vi "Configure Output.vi"(6 "Output Type  (0: Sweeping)":i32(ring) items=["Sweeping", "Measuring", "Main Trigger", "Gate Trigger", "Gate", "Odd/Even Trace Point", "Off"], 8 "error in (no error)":errorcluster, 9 "Trigger Polarity  (0: Positive)":i32(ring) items=["Positive", "Negative"], 10 "Trigger Out  (0: Trigger1)":i32(ring) items=["Trigger1", "Trigger2"], 11 "VISA resource name":refnum<visa-resource-name>) -> (0 "error out":errorcluster, 3 "VISA resource name out":refnum<visa-resource-name>)   [LabVIEW 2018, in "Agilent MXA Series.lvlib"]
doc: "Configures the output signal of the spectrum analyzer."
uses:
  Agilent MXA Series.lvlib
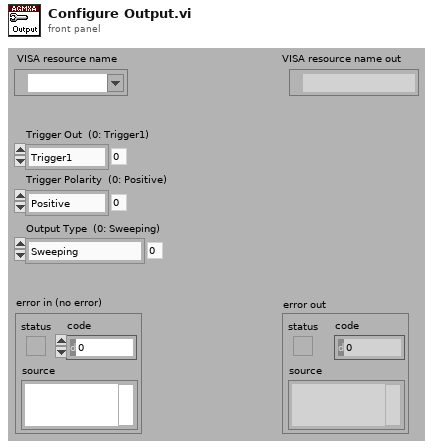
[diagram p1: front panel]
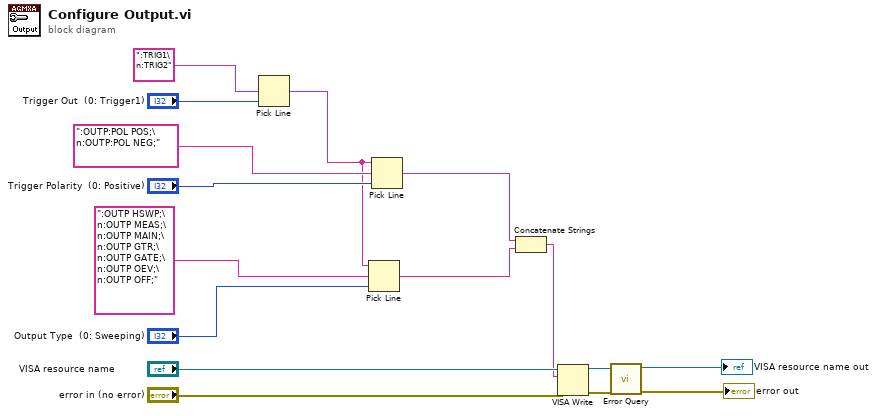
[diagram p0: block diagram]
diagram:
  n1 = Pick Line(multi-line string=":TRIG1\n:TRIG2", line index="Trigger Out  (0: Trigger1)") -> (output string=w2:string)  [unwired: 1 in]
  n2 = Pick Line(string ("")=w2, multi-line string=":OUTP HSWP;\n:OUTP MEAS;\n:OUTP MAIN;\n:OUTP GTR;\n:OUTP GATE;\n:OUTP OEV;\n:OUTP OFF;", line index="Output Type  (0: Sweeping)") -> (output string=w10:string)
  n3 = Pick Line(string ("")=w2, multi-line string=":OUTP:POL POS;\n:OUTP:POL NEG;", line index="Trigger Polarity  (0: Positive)") -> (output string=w1:string)
  n4 = Concatenate Strings(w1, w10) -> (w3:string)
  n5 = VISA Write(VISA resource name="VISA resource name", write buffer=w3, error in (no error)="error in (no error)") -> (VISA resource name out=w6:refnum<visa-resource-name>, error out=w7:errorcluster)  [unwired: 1 out]
  n6 = call "Error Query.vi"("error in (no error)"=w7, "VISA resource name"=w6) -> ("error out"=→"error out":errorcluster, "VISA resource name out"=→"VISA resource name out":refnum<visa-resource-name>)  [unwired: 6 in, 2 out]
